vi "Start Acquisition.vi"(8 "error in (no error)":errorcluster, 10 "Camera Name":string, 11 "Camera in":refnum<class "Camera Actor.lvclass">) -> (0 "error out":errorcluster {"code" format="%.0x"}, 3 "Camera out":refnum<class "Camera Actor.lvclass">)   [LabVIEW 2020, in "Camera Actor.lvlib" / "Camera Actor.lvclass"]
uses:
  Camera Actor.lvclass
  Operation Mode.ctl
  Camera Actor.lvclass/Camera Actor.ctl
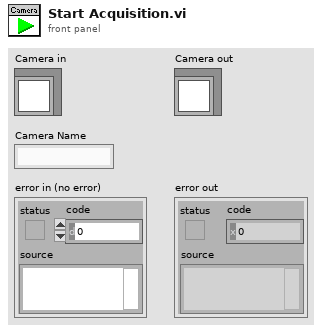
[diagram p1: front panel]
types:
  T1 = typedef "Camera Actor.lvlib/Camera Actor.lvclass/Operation Mode.ctl" = enum16{"Run", "Stop", "Exit", "Error", "Restart"}
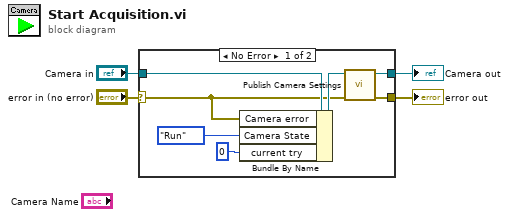
[diagram p0: block diagram]
diagram:
  n1 = case shown="No Error" "error in (no error)" {
    selector: "error in (no error)" -> [w5 w12]
    tunnel: "Camera in" -> [w11 w13]
    tunnel: [w7 w13] -> w3
    tunnel: [w6 w12] -> w1
    frame No Error {
      n2 = Bundle By Name(cluster=w11, "Camera error"=w5, "Camera State"=Operation_Mode."Run", "current try"=u8 0) -> (w10:refnum<class "Camera Actor.lvclass">)
      n3 = call-dynamic "Publish Camera Settings.vi"("error in (no error)"=w5, "Camera Actor in"=w10) -> ("error out"=w6:errorcluster, "Camera Actor out"=w7:refnum<class "Camera Actor.lvclass">)  [unwired: 8 in]
    }
    frame Error {
    }
  }
  "error out" <- w1
  "Camera out" <- w3
